vi "Write Setpoint.vi"(0 "Session Handle":T1, 5 "Setpoint":dbl=10.0 format="%#_13g", 11 "error in (no error)":errorcluster) -> (4 "Session Handle Out":T1, 15 "error out":errorcluster)   [LabVIEW 2015, in "Peltier.lvclass"]
uses:
  Peltier.lvclass
  Typedefs/Session Handle.ctl
  Gas/Gas.lvclass
panel:
  out "Success?":bool
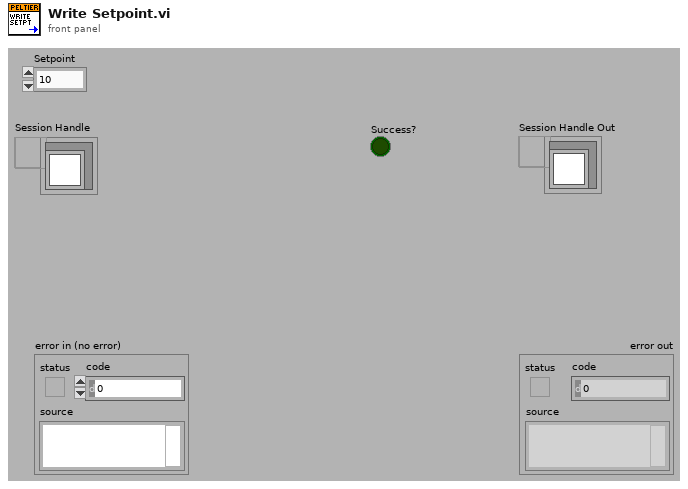
[diagram p1: front panel]
types:
  T1 = typedef "Peltier.lvclass/Session Handle.ctl" = refnum<data-value>
  T2 = typedef "XNET Frame CAN.ctl" = cluster{"timestamp":timestamp, "payload":u8[], "identifier":u32, "type":T3, "extended?":bool, "echo?":bool}
  T3 = typedef "XNET Frame Type CAN.ctl" = u8
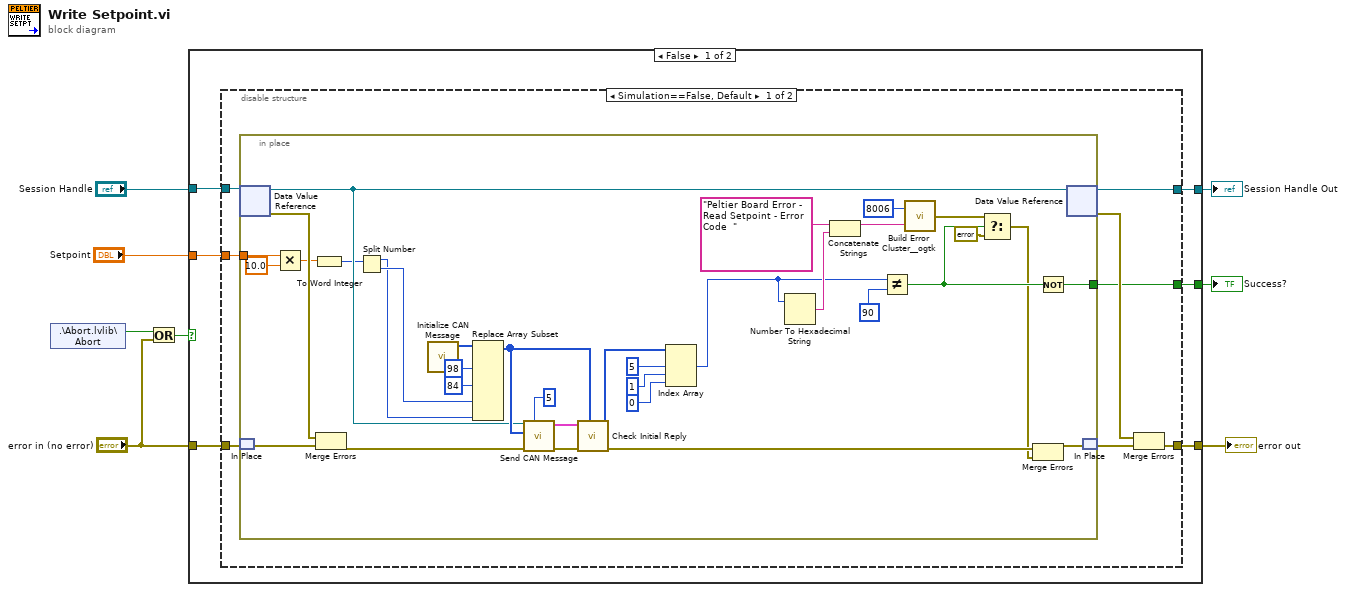
[diagram p0: block diagram]
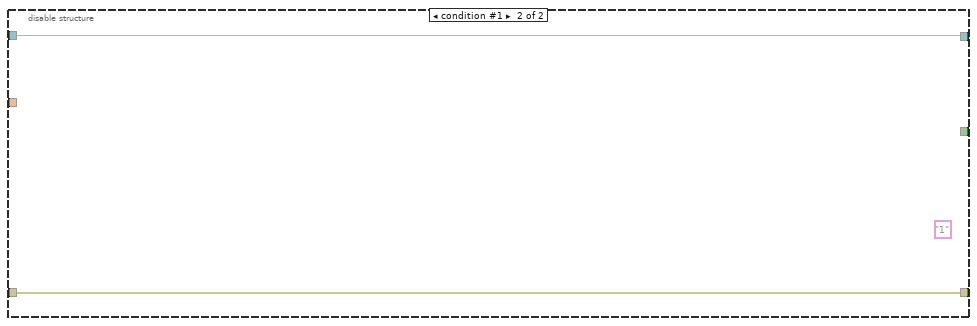
[diagram p2: hidden frame]
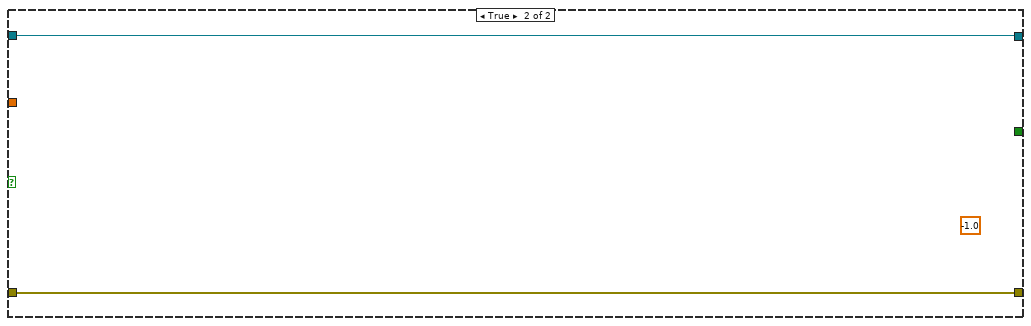
[diagram p3: hidden frame]
diagram:
  n1 = shared-variable ".\\Abort.lvlib\\Abort"() -> (w7:bool)  [unwired: 1 in, 1 out]
  n2 = Or(x=w7, y="error in (no error)") -> (x .or. y?=w5:bool)
  n3 = case shown="False" w5 {
    tunnel: [w14 w60] -> w2
    tunnel: [w13 w59] -> w8
    tunnel: "Session Handle" -> [w12 w60]
    tunnel: "error in (no error)" -> [w11 w59]
    tunnel: [w10 _] -> w4
    tunnel: "Setpoint" -> [w9 _]
    frame False {
      n4 = disable-structure shown="Simulation==False, Default" {
        disable-tunnel: [w22 w58] -> w14
        disable-tunnel: [w19 w57] -> w13
        disable-tunnel: w12 -> [w18 w58]
        disable-tunnel: w11 -> [w17 w57]
        disable-tunnel: [w16 _] -> w10
        disable-tunnel: w9 -> [w15 _]
        frame condition #0 (active) {
          n5 = in-place {
            in-place-border: [w38] -> w16
            in-place-border: w15 -> [w31]
            n6 = in-place-dvr #1(w18) -> (w47:refnum<class "Peltier.lvclass">, w52:errorcluster)
            n7 = in-place-match #2(w17) -> (w51:errorcluster)
            n8 = Multiply(x=w31, y=10.0) -> (x*y=w29:dbl)
            n9 = To Word Integer(number=w29) -> (16bit integer=w28:i16)
            n10 = Merge Errors(w52, w51) -> (w46:errorcluster)
            n11 = Split Number(x=w28) -> (hi(x)=w26:u8, lo(x)=w27:u8)
            n12 = call "Initialize CAN Message.vi"() -> ("Initial Payload"=w54:u8[])  [unwired: 11 in]
            n13 = Replace Array Subset(array=w54, new element #1=u8 98 ("new element/subarray"), new element #2=u8 84 ("new element/subarray"), new element #3=w27, new element #4=w26) -> (w50:u8[])  [unwired: 4 in]
            n14 = call "Send CAN Message.vi"("Number of Retries"=5, "error in (no error)"=w46, "payload"=w50, "Peltier In"=w47) -> ("error out"=w25:errorcluster, "Reply"=w48:T2[])  [unwired: 5 in, 1 out]
            n15 = call "Check Initial Reply.vi"("Write Message"=w50, "error in (no error)"=w25, "Reply"=w48) -> ("error out"=w24:errorcluster, "Data Packet"=w53:u8[])  [unwired: 5 in, 2 out]
            n16 = Index Array(array=w53, index #1=5 ("index"), index #2=1 ("index"), index #3=0 ("index")) -> (element #1=w39:u8)  [unwired: 2 out]
            n17 = Number To Hexadecimal String(2:w39) -> (0:w43:string)  [unwired: 1 in]
            n18 = Concatenate Strings("Peltier Board Error -  Read Setpoint - Error Code  " ("string"), w43) -> (w42:string)
            n19 = Not Equal?(x=w39, y=u8 90 ("new element/subarray")) -> (x != y?=w33:bool)
            n20 = call <userlib>:"Build Error Cluster__ogtk.vi"("String to Prepend to source (\"\")"=w42, "code"=8006) -> ("error out"=w35:errorcluster)
            n21 = Select(t=w35, s=w33, f=errorcluster {"status"=FALSE, "code"=0, "source"=""}) -> (s? t:f=w23:errorcluster)
            n22 = Merge Errors(w24, w23) -> (w55:errorcluster)
            n23 = Not(x=w33) -> (.not. x?=w38:bool)
            n24 = in-place-dvr #1(w47) -> (w22:T1, w20:errorcluster)
            n25 = in-place-match #2(w55) -> (w21:errorcluster)
          }
          n26 = Merge Errors(w20, w21) -> (w19:errorcluster)
        }
        frame condition #1 {
          (unwired) "1"
        }
      }
    }
    frame True {
      (unwired) -1.0
    }
  }
  "error out" <- w8
  "Success?" <- w4
  "Session Handle Out" <- w2
